vi "Drawing.vi"() -> ()   [LabVIEW 2021]
uses:
  <vilib>/Utility/inputDevices.llb/mouseAcquire.vi
  <vilib>/Utility/inputDevices.llb/closeMouse.vi
panel:
  in  "Cancel Drawing Queue":bool
  out "Robot Drawn So Far":cluster{"X":dbl, "Y":dbl}[](graph)
  out "Obstacle Detected":bool
  out "Robot Vertical":dbl
  out "Robot Horizontal":dbl
  out "Chalk Force Readout":dbl
  in  "Clear Drawing Plane":bool
  out "Current Mouse Coordinates":T1
  out "Drawing":cluster{i32[], i32[]}[](graph)
  out "Mouse Status":cluster{"Clicked?":bool}
  in  "Emergency Stop":bool
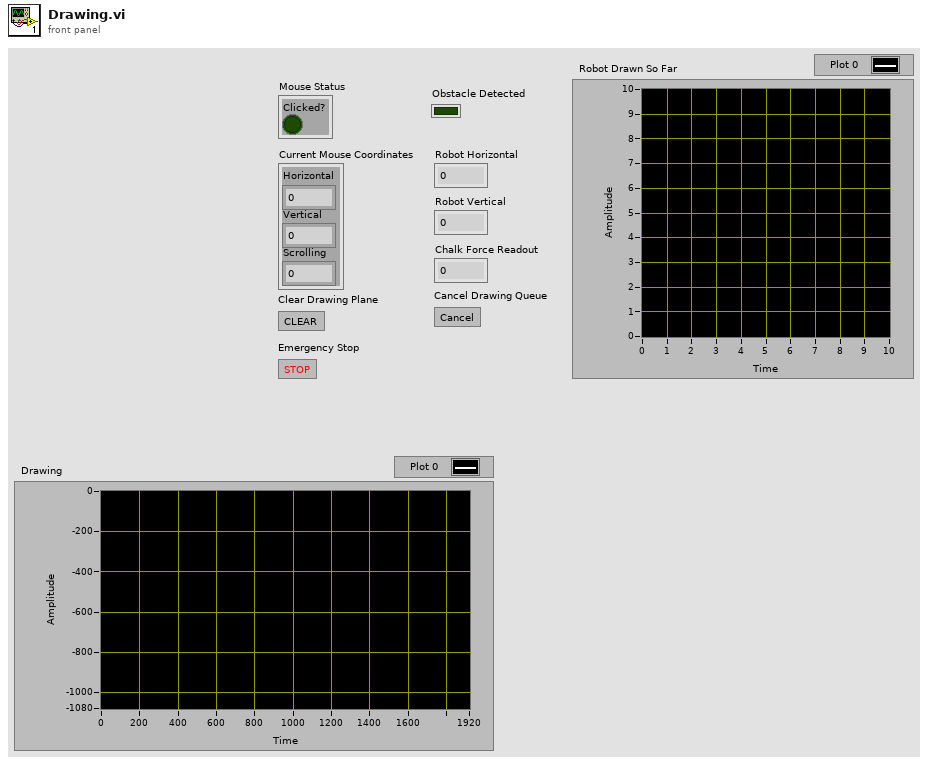
[diagram p1: front panel]
types:
  T1 = cluster{"Horizontal":i32, "Vertical":i32, "Scrolling":i32}
  T2 = cluster{"button 1":bool, "button 2":bool, "button 3":bool, "button 4":bool}
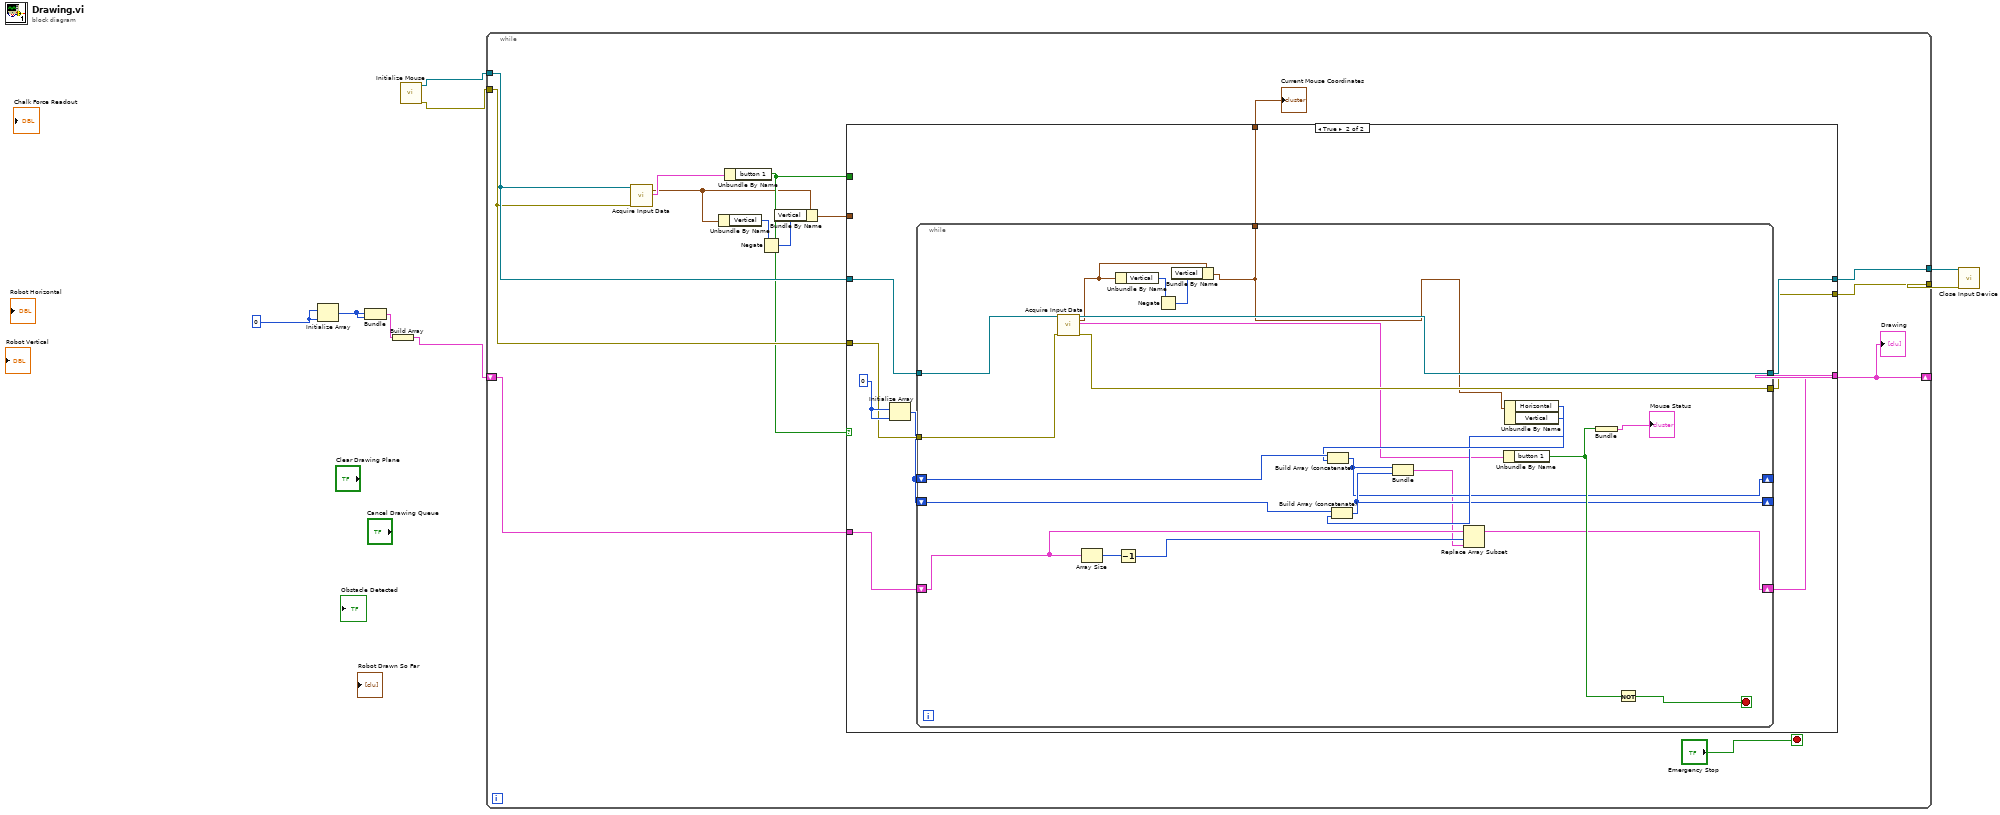
[diagram p0: block diagram]
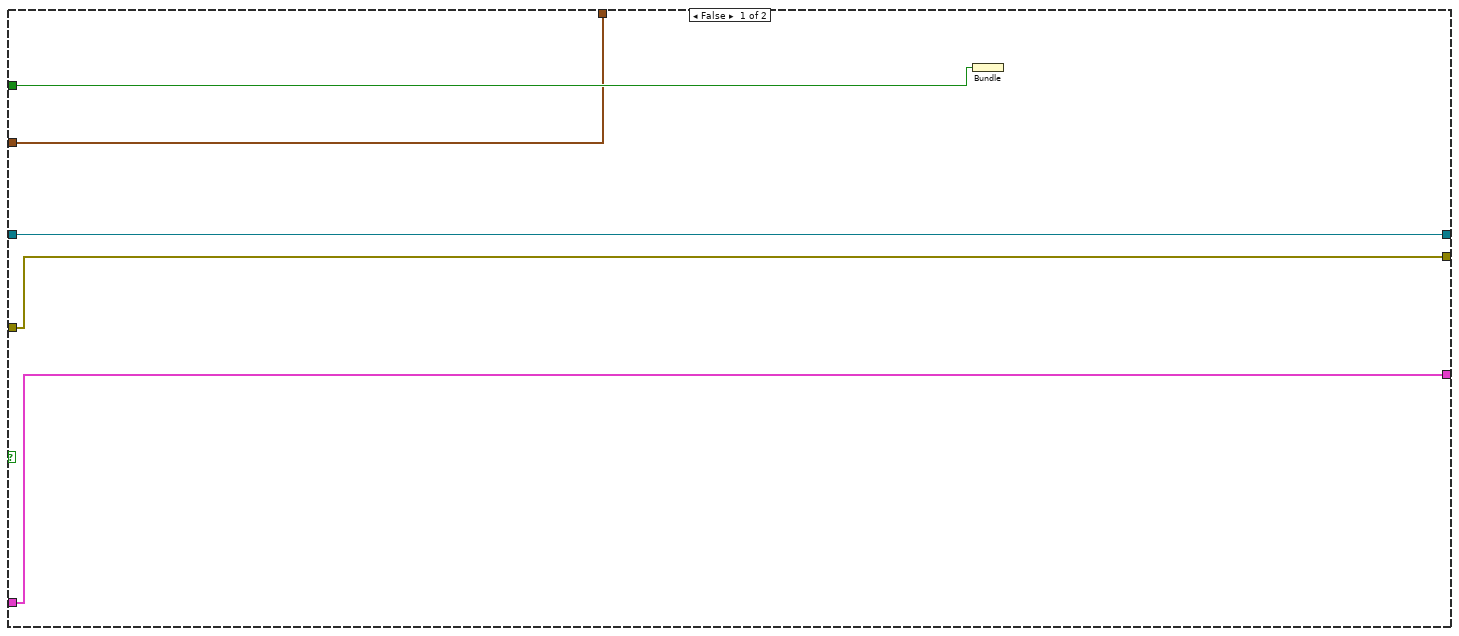
[diagram p2: hidden frame]
diagram:
  w6 = 0
  n1 = Initialize Array(w6, w6) -> (w5:i32[])
  n2 = Bundle(w5, w5) -> (w4:cluster{i32[], i32[]})  [unwired: 1 in]
  n3 = Build Array(w4) -> (w3:cluster{i32[], i32[]}[])
  n4 = call <vilib>:"Initialize Mouse.vi"() -> ("error out"=w7:errorcluster, "device ID"=w8:refnum<k1>)  [unwired: 10 in]
  n5 = while {
    tunnel: w8 -> [w17]
    tunnel: w7 -> [w16]
    shift-right: [w9] -> _
    shift-left: w3 -> [w21]
    tunnel: [w20] -> w2
    tunnel: [w19] -> w1
    stop <- "Emergency Stop" stop-if-true
    n6 = call-poly <vilib>:"Acquire Input Data.vi"("device ID"=w17, "error in (no error)"=w16) -> ("axis info"=w13:T1, "button info"=w15:T2)  [unwired: 14 in, 2 out]
    n7 = Unbundle By Name(w13) -> ("Vertical"=w12:i32)
    n8 = Unbundle By Name(w15) -> ("button 1"=w14:bool)
    n9 = Negate(x=w12) -> (-x=w11:i32)
    n10 = Bundle By Name(cluster=w13, "Vertical"=w11) -> (w10:T1)
    n11 = case shown="True" w14 {
      tunnel: w21 -> [w23 w36]
      tunnel: [w23 w28] -> w9
      tunnel: w16 -> [w27 w34]
      tunnel: w17 -> [w26 w32]
      tunnel: [w26 w31] -> w20
      tunnel: [w27 w30] -> w19
      tunnel: [w24 w29] -> w18
      tunnel: w14 -> [w25 _]
      tunnel: w10 -> [w24 _]
      frame False {
        n12 = Bundle("button 1"=w25) -> ()  [unwired: 1 in, 1 out]
      }
      frame True {
        w35 = 0
        n13 = Initialize Array(w35, w35) -> (w33:i32[])
        n14 = while {
          shift-right: [w37] -> w28
          shift-left: w36 -> [w39]
          shift-right: [w47] -> _
          shift-left: w33 -> [w58]
          shift-right: [w48] -> _
          shift-left: w33 -> [w57]
          tunnel: w34 -> [w56]
          tunnel: w32 -> [w53]
          tunnel: [w52] -> w31
          tunnel: [w51] -> w30
          tunnel: [w43] -> w29
          stop <- w59 stop-if-true
          n15 = call-poly <vilib>:"Acquire Input Data.vi"("device ID"=w53, "error in (no error)"=w56) -> ("device ID"=w52:refnum<k1>, "axis info"=w44:T1, "button info"=w50:T2, "error out"=w51:errorcluster)  [unwired: 14 in]
          n16 = Array Size(array=w39) -> (size(s)=w41:i32)
          n17 = Unbundle By Name(w44) -> ("Vertical"=w46:i32)
          n18 = Decrement(x=w41) -> (x-1=w40:i32)
          n19 = Negate(x=w46) -> (-x=w45:i32)
          n20 = Bundle By Name(cluster=w44, "Vertical"=w45) -> (w43:T1)
          n21 = Unbundle By Name(w50) -> ("button 1"=w49:bool)
          n22 = Unbundle By Name(w43) -> ("Horizontal"=w55:i32, "Vertical"=w54:i32)
          n23 = Build Array (concatenate)(w58, w55) -> (w47:i32[])
          n24 = Build Array (concatenate)(w57, w54) -> (w48:i32[])
          n25 = Bundle(w47, w48) -> (w38:cluster{i32[], i32[]})  [unwired: 1 in]
          n26 = Replace Array Subset(array=w39, new element=w38, index=w40) -> (w37:cluster{i32[], i32[]}[])
          n27 = Bundle("button 1"=w49) -> (→"Mouse Status":cluster{"button 1":bool})  [unwired: 1 in]
          n28 = Not(x=w49) -> (.not. x?=w59:bool)
        }
      }
    }
    "Current Mouse Coordinates" <- w18
    "Drawing" <- w9
  }
  n29 = call-poly <vilib>:"Close Input Device.vi"("error in (no error)"=w1, "device ID"=w2) -> ()  [unwired: 8 in, 1 out]
